vi "RT - Send Message to UI.vi"(8 "error in (no error)":errorcluster caption="错误输入（无错误）", 9 "Message Data":variant caption="消息数据", 10 "Message":string caption="消息") -> (0 "error out":errorcluster caption="错误输出")   [LabVIEW 2013]
uses:
  Message Queue/Message Cluster.ctl
  Globals/Global - RT Stream Connections.vi
  Globals/Global - Configuration Options.vi
  Message Queue/Message Queue.lvlib
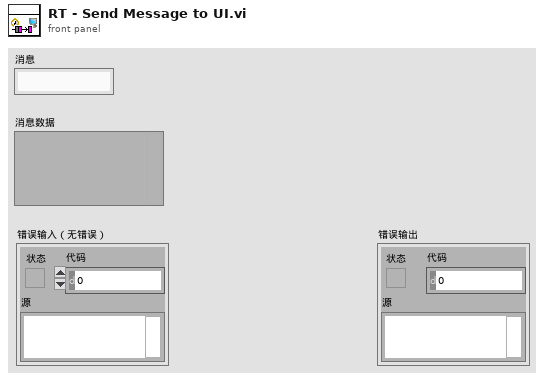
[diagram p1: front panel]
types:
  T1 = typedef "Message Queue.lvlib/Message Cluster.ctl" = cluster{"Message":string, "Message Data":variant}
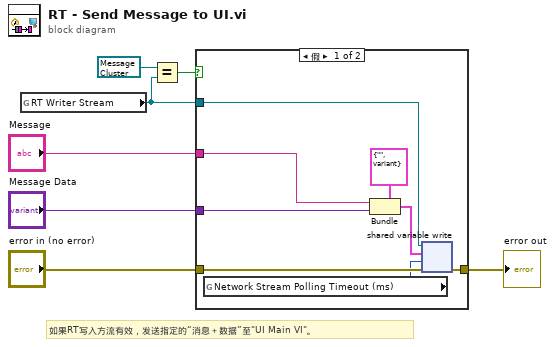
[diagram p0: block diagram]
diagram:
  # "如果RT写入方流有效，发送指定的“消息＋数据”至\"UI Main VI\"。"
  n1 = global read "Global - RT Stream Connections.vi" "RT Writer Stream"() -> (w1:refnum<k21>)
  n2 = Equal?(x=refnum<k21> refnum ("RT Writer Stream"), y=w1) -> (x = y?=w5:bool)
  n3 = case shown="假" w5 {
    tunnel: [w15 w16] -> w2
    tunnel: "error in (no error)" -> [w14 w16]
    tunnel: "Message Data" -> [w13 _]
    tunnel: w1 -> [w11 _]
    tunnel: "Message" -> [w9 _]
    frame False {
      n4 = global read "Global - Configuration Options.vi" "Network Stream Polling Timeout (ms)"() -> (w8:i32)
      n5 = Bundle(cluster=T1 {"Message"="", "Message Data"=variant} ("Message Cluster"), "Message"=w9, "Message Data"=w13) -> (w12:T1)
      n6 = shared-variable-write(w11, w14, w12, w8) -> (w15:errorcluster)  [unwired: 2 out]
    }
    frame True {
    }
  }
  "error out" <- w2
